vi "Configure List Step.vi"(6 "List Timer":i32=1 min=0, 7 "List Index":i32=1 min=1, 8 "error in (no error)":errorcluster, 9 "Trigger Current Limit (0.0 A)":dbl format="%.2g", 10 "Trigger Voltage Limit (0.0 V)":dbl format="%.2g", 11 "VISA resource name":refnum<visa-resource-name>) -> (0 "error out":errorcluster, 3 "VISA resource name out":refnum<visa-resource-name>)   [LabVIEW 2015, in "IT6700H.lvlib"]
uses:
  <instrlib>/IT6700H/IT6700H.lvlib
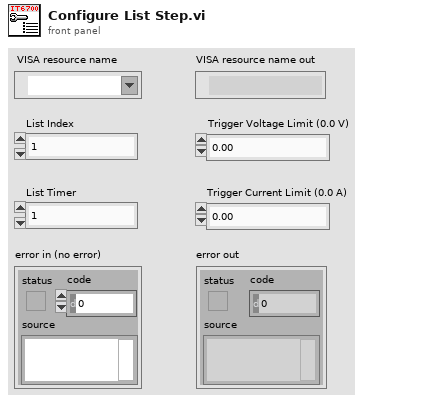
[diagram p1: front panel]
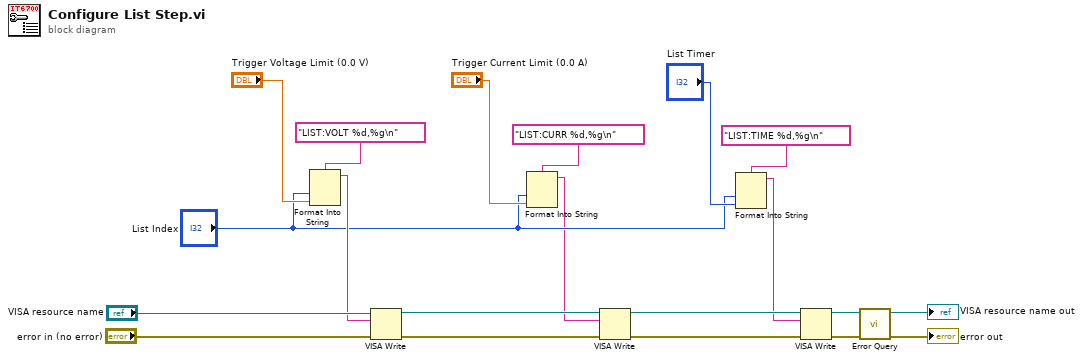
[diagram p0: block diagram]
diagram:
  n1 = Format Into String(format string="LIST:VOLT %d,%g\n", "List Index", "Trigger Voltage Limit (0.0 V)") -> (resulting string=w12:string)  [unwired: 2 in, 1 out]
  n2 = VISA Write(VISA resource name="VISA resource name", write buffer=w12, error in (no error)="error in (no error)") -> (VISA resource name out=w6:refnum<visa-resource-name>, error out=w4:errorcluster)  [unwired: 1 out]
  n3 = Format Into String(format string="LIST:CURR %d,%g\n", "List Index", "Trigger Current Limit (0.0 A)") -> (resulting string=w2:string)  [unwired: 2 in, 1 out]
  n4 = VISA Write(VISA resource name=w6, write buffer=w2, error in (no error)=w4) -> (VISA resource name out=w5:refnum<visa-resource-name>, error out=w3:errorcluster)  [unwired: 1 out]
  n5 = Format Into String(format string="LIST:TIME %d,%g\n", "List Index", "List Timer") -> (resulting string=w1:string)  [unwired: 2 in, 1 out]
  n6 = VISA Write(VISA resource name=w5, write buffer=w1, error in (no error)=w3) -> (VISA resource name out=w17:refnum<visa-resource-name>, error out=w18:errorcluster)  [unwired: 1 out]
  n7 = call <instrlib>:"Error Query.vi"("error in (no error)"=w18, "VISA resource name"=w17) -> ("error out"=→"error out":errorcluster, "VISA resource name out"=→"VISA resource name out":refnum<visa-resource-name>)  [unwired: 6 in, 2 out]
